vi "mlink_dsp_mem_write.vi"(8 "error in (no error)":errorcluster, 9 "data":sgl[](array[numeric]), 10 "start index":i32=1, 11 "connection ID":i32=-1) -> (0 "error put":errorcluster, 3 "connection ID out":i32)   [LabVIEW 2009, in "MicroDAQ.lvlib" / "mlink.lvlib"]
doc: "This function allows writing user data to DSP application during its execution. The function has to be used with Xcos MEM read block. Function writes data from start_idx to start_inx + len. MEM read block can read up to 250000 values."
uses:
  <instrlib>/MicroDAQ/Mlink library wraper/mlink.lvlib
  <instrlib>/MicroDAQ/MLink32.dll
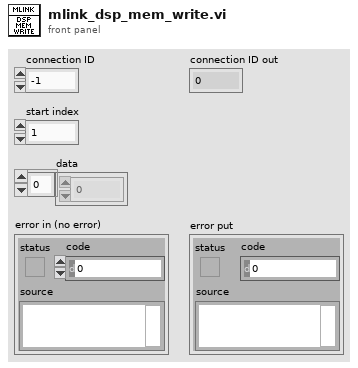
[diagram p1: front panel]
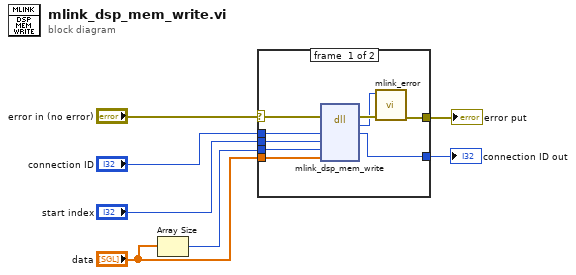
[diagram p0: block diagram]
diagram:
  n1 = Array Size(array="data") -> (size(s)=w4:i32)
  n2 = case shown="No Error" "error in (no error)" {
    selector: "error in (no error)" -> [w11 w18]
    tunnel: "connection ID" -> [w16 w17]
    tunnel: "start index" -> [w15 _]
    tunnel: "data" -> [w14 _]
    tunnel: w4 -> [w13 _]
    tunnel: [w12 w17] -> w3
    tunnel: [w8 w18] -> w1
    frame #0 {
      n3 = dll-call lib="C:/Program Files (x86)/National Instruments/LabVIEW 2009/instr.lib/MicroDAQ/MLink32.dll" fn="mlink_dsp_mem_write"(error in=w11, "link_fd"=w16, "start_idx"=w15, "len"=w13, "data"=w14) -> (error out=w10:errorcluster, "return type"=w9:i32, "link_fd"=w12:i32)  [unwired: 5 in, 1 out]
      n4 = call <instrlib>:"mlink_error.vi"("error in (no error)"=w10, "error code"=w9) -> ("error out"=w8:errorcluster)  [unwired: 9 in]
    }
    frame #1 {
    }
  }
  "connection ID out" <- w3
  "error put" <- w1
